vi "FPGAmain_5772.vi"() -> ()   [LabVIEW 2013]
uses:
  FPGA/DataMode.ctl
  FPGA/AcquireState.ctl
  <vilib>/Platform/TimedLoop/XDataNode/timing_clust.ctl
  <vilib>/Platform/TimedLoop/XDataNode/nitl_modes.ctl
  <vilib>/Platform/TimedLoop/XDataNode/wakeup.ctl
  <vilib>/rvi/Emulation/niFpgaSctlEmulationGetInTimedLoop.vi
  <vilib>/rvi/Emulation/niFpgaEmulationReportErrorSimple.vi
  <vilib>/rvi/Emulation/niFpgaGetClockAttributes.vi
  <vilib>/rvi/Emulation/niFpgaCriticalErrorInLSC.vi
  <vilib>/rvi/FIFO/Fifo_Resource/nirvififoEmulationReadFpgaImpl.vi
  <vilib>/rvi/DataTransferAndStorage/Container/Common/niFpgaContainerGetUniqueNameForEmu.vi
  <vilib>/rvi/Emulation/niFpgaProcessEmulError.vi
  <vilib>/rvi/interface/RandomDataEmulation/nirviRandomDataFPGAFIFO.vi
  <vilib>/rvi/interface/RandomDataEmulation/niFpgaRandomDataHandleErrors.vi
  <vilib>/rvi/eio/common/nirviEmuTemplateMethod_errors.vi
  <vilib>/rvi/FIFO/Fifo_Resource/nirvififoEmulationWriteFpgaImpl.vi
  <vilib>/Platform/TimedLoop/XDataNode/XDataNode.xnode
  <vilib>/rvi/DataTransferAndStorage/Container/XNode/niFpgaContainer.xnode
  <vilib>/rvi/FIFO/Fifo_Resource/nirvififoEmulationRead.vi
  <vilib>/rvi/interface/RandomDataEmulation/nirviRandomDataFpgaReadWriteTemplate.vi
  <vilib>/eio/EIONode/EIONode.xnode
  <vilib>/rvi/FIFO/Fifo_Resource/nirvififoEmulationWrite.vi
  <vilib>/Platform/TimedLoop/XDataNode/XDNodeRunTimeDep.lvlib
panel:
  in  "Simulated phase":fxp<+,64,64>[](array[numeric])=[0.0, 0.0, 0.0, 0.0]
  in  "Acquisition running":bool
  out "DMA Timed Out?":bool
  in  "Phase":fxp<+,64,64>[](array[numeric])=[0.0, 0.0, 0.0, 0.0]
  in  "Trigger Acquisition":bool
  in  "Mode":T1
  in  "Samples Per Trigger":u64=128000 min=1 step=1
  in  "User Command Commit":bool
  in  "User Command":u8
  out "User Command Idle":bool
  out "User Command Status":u8
  in  "User Data 0":u16
  in  "User Data 1":u8
  out "PLL Locked":bool
  out "User Error":bool
  out "Configured?":bool
  # "Configuration"
  # "Aqcuistion"
  # "Simulated IQ"
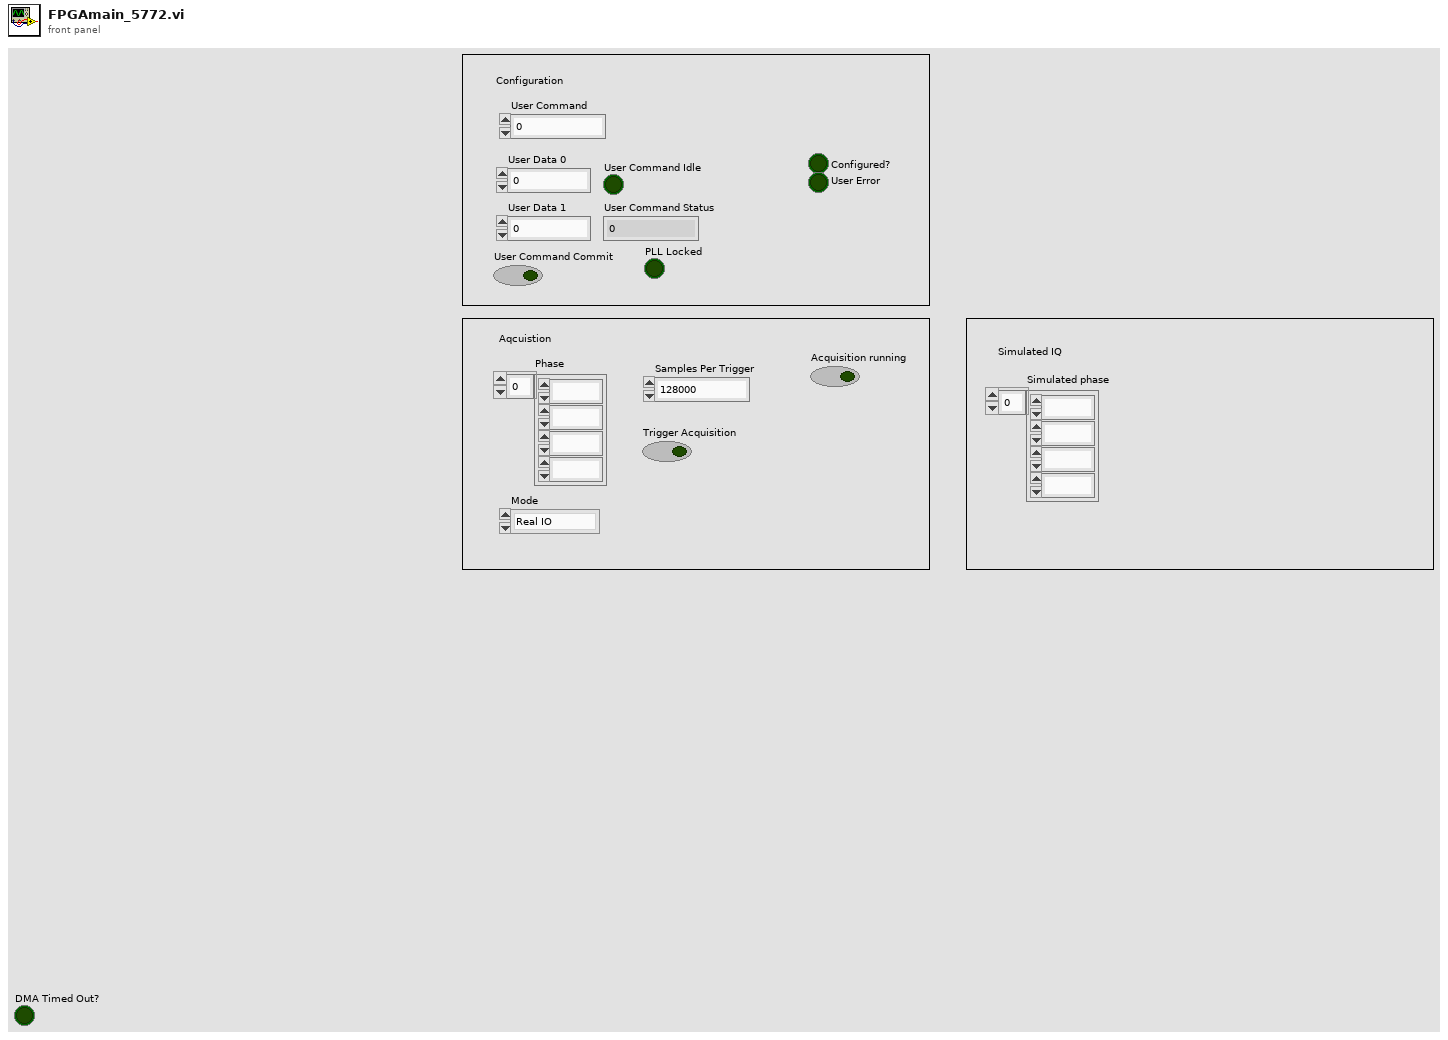
[diagram p1: front panel]
types:
  T1 = typedef "DataMode.ctl" = enum16{"Real IO", "Simulated"}
  T2 = typedef "AcquireState.ctl" = enum8{"Idle", "Acquire"}
  T3 = typedef "XDNodeRunTimeDep.lvlib/timing_clust.ctl" = cluster{"Expected End [f-1]":u64, "Actual End [f-1]":u64, "Finished Late? [f-1]":bool, "Expected End [i-1]":u64, "Actual End [i-1]":u64, "Finished Late? [i-1]":bool, "Expected Start [i]":u64, "Actual Start [i]":u64, "Expected Start [f]":u64, "Actual Start [f]":u64, "Source Name":string, "Structure Name":string, "Period":i64, "Deadline":i64, "Offset":i64, "Start":i64, "Priority":i32, "Timeout":i32, "Mode":T4, "Wakeup Reason":T5, "Error":errorcluster, "Source Type":string, "Secondary Source Type":string, "Global End Time":u64, "Global Start Time":u64, "Frame Duration":u64, "Iteration Duration":u64, "Assigned CPU":i32, "I/O Scan Engine Mode":u32}
  T4 = typedef "XDNodeRunTimeDep.lvlib/nitl_modes.ctl" = enum32{"No Change", "Process missed periods, maintain original phase", "Discard missed periods, maintain original phase", "Process missed periods, ignore original phase", "Discard missed periods, ignore original phase"}
  T5 = typedef "XDNodeRunTimeDep.lvlib/wakeup.ctl" = enum32{"Normal", "Aborted", "Asynchronous wakeup", "Timing source error", "Timed loop error", "Timeout"}
  T6 = typedef "I16 array size 4.ctl" = i16[]
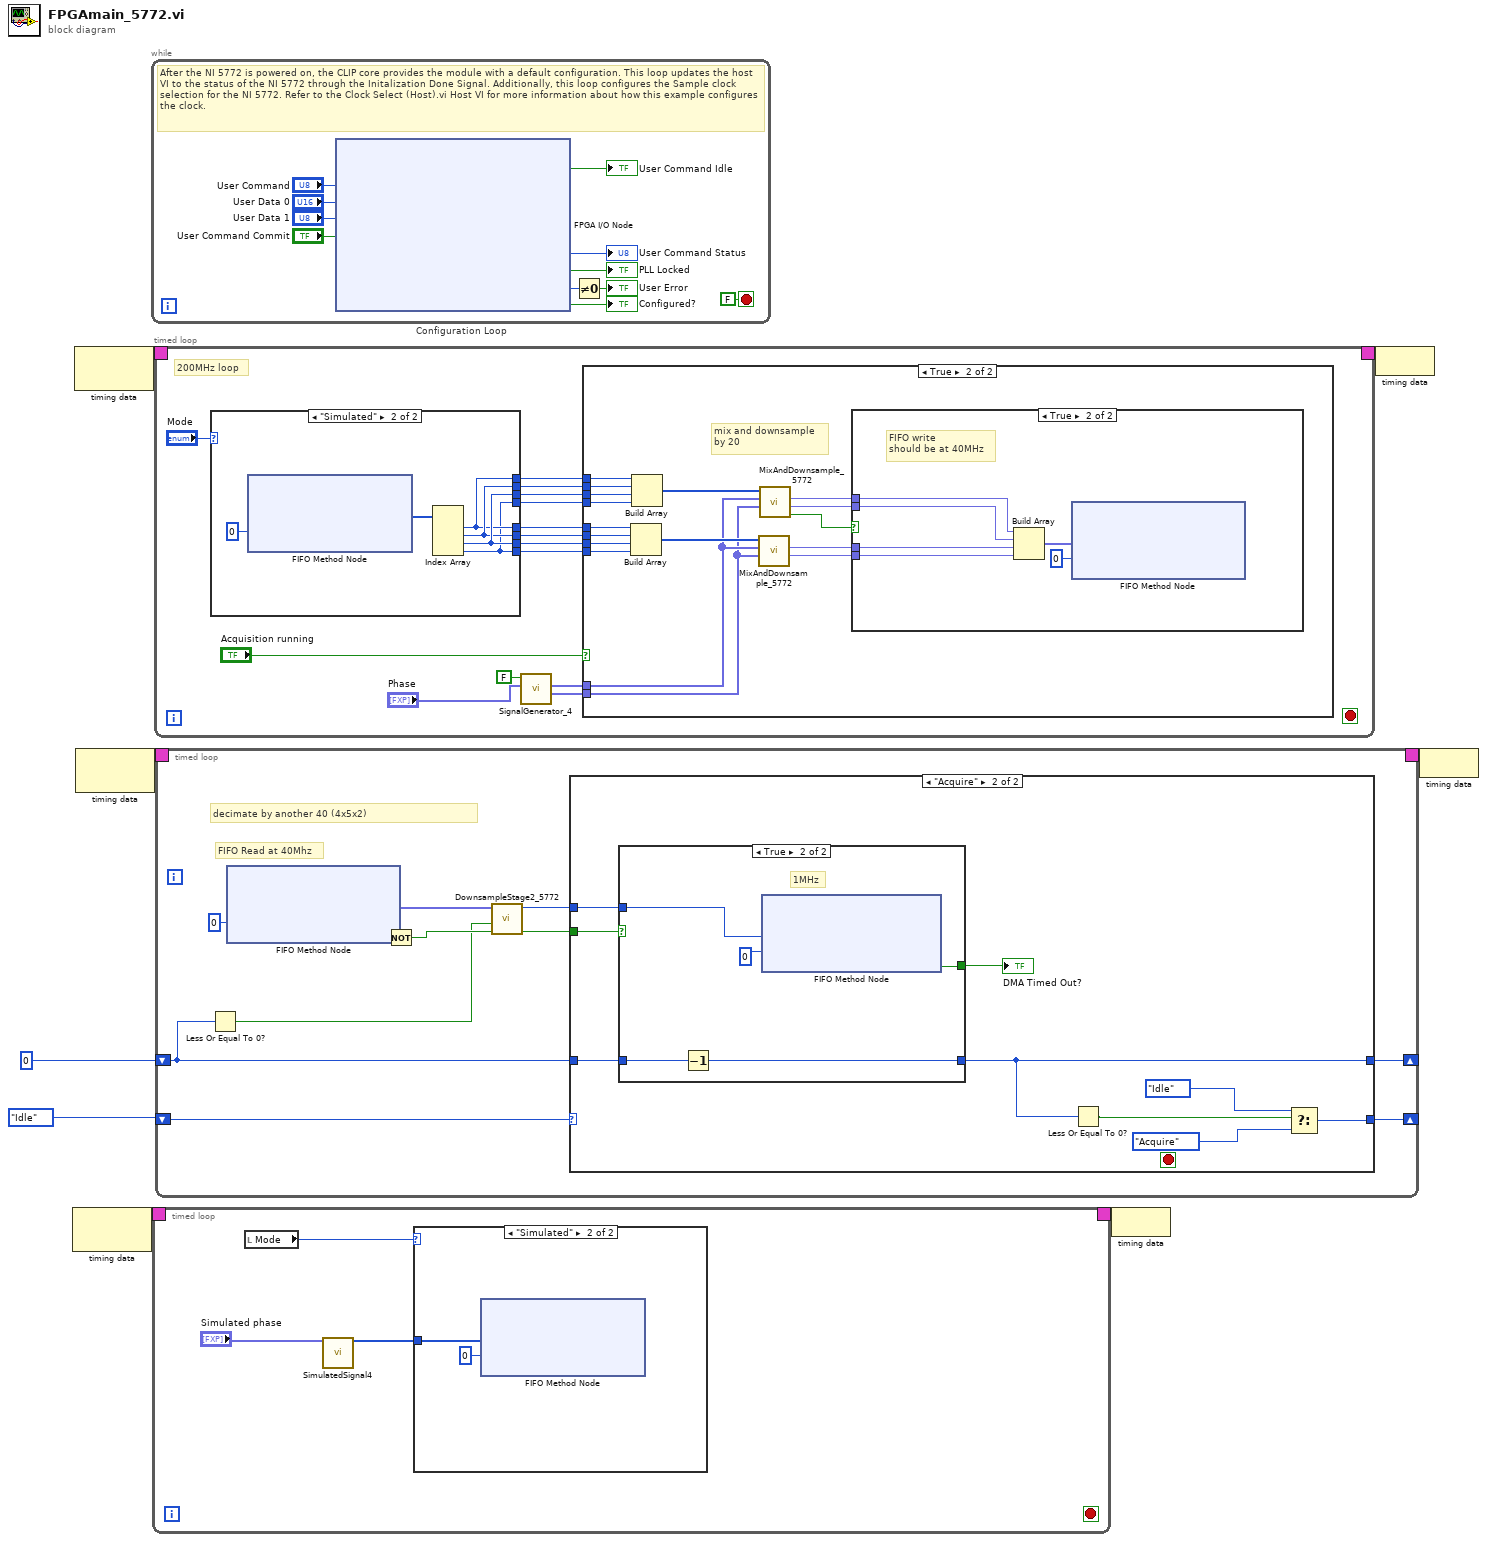
[diagram p0: block diagram]
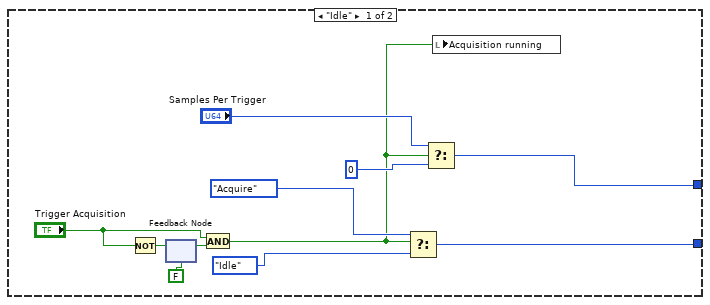
[diagram p3: hidden frame]
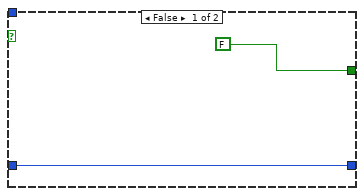
[diagram p4: hidden frame]
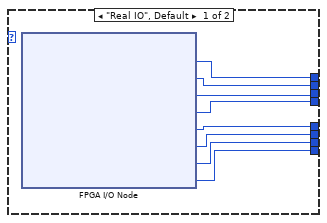
[diagram p7: hidden frame]
diagram:
  n1 = node-c288() -> (w4:T3)  [unwired: 1 in]
  n2 = node-c288() -> (w8:T3)  [unwired: 1 in]
  n3 = node-c288() -> (w6:T3)  [unwired: 1 in]
  n4 = while "Configuration Loop" {
    stop <- FALSE stop-if-true
    # "After the NI 5772 is powered on, the CLIP core provides the module with a default configuration. This loop updates the host VI to the status of the NI 5772 through the Initalization Done Signal. Additionally, this loop configures the Sample clock selection for the NI 5772. Refer to the Clock Select (Host).vi Host VI for more information about how this example configures the clock."
    n5 = xnode "FPGA I/O Node"("IO Module\\User Command"="User Command", "IO Module\\User Data 0"="User Data 0", "IO Module\\User Data 1"="User Data 1", "IO Module\\User Command Commit"="User Command Commit") -> ("IO Module\\User Command Idle"=→"User Command Idle":bool, "IO Module\\User Command Status"=→"User Command Status":u8, "IO Module\\PLL Locked"=→"PLL Locked":bool, "IO Module\\User Error"=w14:u8, "IO Module\\Initialization Done"=→"Configured?":bool)  [unwired: 9 in, 9 out]
    n6 = Not Equal To 0?(x=w14) -> (x != 0?=→"User Error":bool)
  }
  n7 = timed-loop {
    timing: w4 -> [_]
    timing-out: [_] -> w3
    stop <- _ stop-if-true
    n8 = local read "Mode"() -> (w22:T1)
    n9 = call "SimulatedSignal4.vi"("Phase"="Simulated phase") -> ("output"=w21:T6)  [unwired: 9 in, 1 out]
    n10 = case shown="\"Simulated\"" w22 {
      tunnel: w21 -> [_ w23]
      frame "Real IO", Default {
      }
      frame "Simulated" {
        n11 = xnode ("FIFO Method Node")("Element"=w23, "Timeout"=0) -> ()  [unwired: 1 in, 2 out]
      }
    }
  }
  n12 = timed-loop {
    timing: w8 -> [_]
    timing-out: [_] -> w7
    stop <- _ stop-if-true
    # "200MHz loop"
    n13 = case shown="\"Simulated\"" "Mode" {
      tunnel: [w71 w73] -> w40
      tunnel: [w70 w74] -> w39
      tunnel: [w69 w75] -> w38
      tunnel: [w68 w72] -> w37
      tunnel: [w67 w73] -> w35
      tunnel: [w66 w74] -> w34
      tunnel: [w65 w72] -> w33
      tunnel: [w64 w75] -> w32
      frame "Real IO", Default {
        n14 = xnode "FPGA I/O Node"() -> ("IO Module\\AI 0 Data N-3"=w71:i16, "IO Module\\AI 0 Data N-2"=w70:i16, "IO Module\\AI 0 Data N-1"=w69:i16, "IO Module\\AI 0 Data N"=w68:i16, "IO Module\\AI 1 Data N-3"=w67:i16, "IO Module\\AI 1 Data N-2"=w66:i16, "IO Module\\AI 1 Data N-1"=w64:i16, "IO Module\\AI 1 Data N"=w65:i16)  [unwired: 8 in, 8 out]
      }
      frame "Simulated" {
        n15 = xnode ("FIFO Method Node")("Timeout"=0) -> ("Element"=w76:i16[])  [unwired: 1 in, 2 out]
        n16 = Index Array(array=w76) -> (element #1=w73:i16, element #2=w74:i16, element #3=w75:i16, element #4=w72:i16)  [unwired: 4 in]
      }
    }
    n17 = call "SignalGenerator_4.vi"("Phase"="Phase", "reset"=FALSE) -> ("Sine out"=w29:fxp<+/-,16,0>[], "Cosine out"=w30:fxp<+/-,16,0>[])  [unwired: 8 in]
    n18 = case shown="True" "Acquisition running" {
      tunnel: w40 -> [_ w57]
      tunnel: w39 -> [_ w56]
      tunnel: w38 -> [_ w55]
      tunnel: w37 -> [_ w54]
      tunnel: w35 -> [_ w53]
      tunnel: w34 -> [_ w52]
      tunnel: w33 -> [_ w51]
      tunnel: w32 -> [_ w50]
      tunnel: w30 -> [_ w47]
      tunnel: w29 -> [_ w46]
      frame False {
      }
      frame True {
        # "mix and downsample\nby 20"
        n19 = Build Array(w53, w52, w50, w51) -> (w48:i16[])
        n20 = Build Array(w57, w56, w55, w54) -> (w49:i16[])
        n21 = call "MixAndDownsample_5772.vi"("Sine in"=w46, "Cosine in"=w47, "Signal Input"=w48) -> ("Q out"=w41:fxp<+/-,16,14>, "I out"=w42:fxp<+/-,16,14>)  [unwired: 6 in, 1 out]
        n22 = call "MixAndDownsample_5772.vi"("Sine in"=w46, "Cosine in"=w47, "Signal Input"=w49) -> ("data valid"=w43:bool, "Q out"=w44:fxp<+/-,16,14>, "I out"=w45:fxp<+/-,16,14>)  [unwired: 6 in]
        n23 = case shown="True" w43 {
          tunnel: w44 -> [_ w63]
          tunnel: w45 -> [_ w60]
          tunnel: w42 -> [_ w59]
          tunnel: w41 -> [_ w58]
          frame False {
          }
          frame True {
            # "FIFO write\nshould be at 40MHz"
            n24 = Build Array(w60, w63, w59, w58) -> (w62:fxp<+/-,16,14>[])
            n25 = xnode ("FIFO Method Node")("Element"=w62, "Timeout"=0) -> ()  [unwired: 1 in, 2 out]
          }
        }
      }
    }
  }
  n26 = timed-loop {
    timing: w6 -> [_]
    timing-out: [_] -> w5
    shift-right: [w83] -> _
    shift-left: AcquireState."Idle" ("Acquire State") -> [w85]
    shift-right: [w82] -> _
    shift-left: u64 0 ("Samples Per Trigger") -> [w84]
    stop <- _ stop-if-true
    # "FIFO Read at 40Mhz"
    # "decimate by another 40 (4x5x2)"
    n27 = Less Or Equal To 0?(x=w84) -> (x <= 0?=w86:bool)
    n28 = xnode ("FIFO Method Node")("Timeout"=0) -> ("Element"=w88:fxp<+/-,16,14>[], "Timed Out?"=w80:bool)  [unwired: 1 in, 1 out]
    n29 = Not(x=w80) -> (.not. x?=w87:bool)
    n30 = call "DownsampleStage2_5772.vi"("valid in"=w87, "reset"=w86, "Element"=w88) -> ("valid out"=w89:bool, "Element"=w90:u64)  [unwired: 7 in]
    n31 = case shown="\"Acquire\"" w85 {
      tunnel: w90 -> [_ w109]
      tunnel: w89 -> [_ w108]
      tunnel: w84 -> [_ w104]
      tunnel: [w95 w103] -> w83
      tunnel: [w92 w102] -> w82
      frame "Idle" {
        n32 = Not(x="Trigger Acquisition") -> (.not. x?=w96:bool)
        n33 = feedback #1(FALSE) -> (w97:bool)
        n34 = feedback-in #1(w96) -> ()
        n35 = And(x="Trigger Acquisition", y=w97) -> (x .and. y?=w91:bool)
        n36 = Select(t=AcquireState."Acquire" ("Acquire State"), s=w91, f=AcquireState."Idle" ("Acquire State")) -> (s? t:f=w95:T2)
        n37 = Select(t="Samples Per Trigger", s=w91, f=u64 0) -> (s? t:f=w92:u64)
        n38 = local write "Acquisition running"(w91) -> ()
      }
      frame "Acquire" {
        n39 = case shown="True" w108 {
          tunnel: w109 -> [_ w115]
          tunnel: [FALSE ("Timed Out?") w116] -> w110
          tunnel: w104 -> [w111 w114]
          tunnel: [w111 w113] -> w102
          frame False {
          }
          frame True {
            # "1MHz"
            n40 = Decrement(x=w114) -> (x-1=w113:u64)
            n41 = xnode ("FIFO Method Node")("Element"=w115, "Timeout"=0) -> ("Timed Out?"=w116:bool)  [unwired: 1 in, 1 out]
          }
        }
        "DMA Timed Out?" <- w110
        n42 = Less Or Equal To 0?(x=w102) -> (x <= 0?=w106:bool)
        n43 = Select(t=AcquireState."Idle" ("Acquire State"), s=w106, f=AcquireState."Acquire" ("Acquire State")) -> (s? t:f=w103:T2)
      }
    }
  }
  n44 = node-c288(w3) -> ()
  n45 = node-c288(w7) -> ()
  n46 = node-c288(w5) -> ()
